vi "writeToXML.vi"(8 "error in (no error)":errorcluster, 10 "Class Label":string, 11 "ADCPointingCorrectionOffsets in":refnum<class "ADCPointingCorrectionOffsets.lvclass">) -> (0 "error out":errorcluster, 2 "XML out":string, 3 "ADCPointingCorrectionOffsets out":refnum<class "ADCPointingCorrectionOffsets.lvclass">)   [LabVIEW 2022 SP3, in "TCSDataDefinitions.lvlib" / "TCSAtmosphericDispersionCommand.lvlib" / "ADCPointingCorrectionOffsets.lvclass"]
uses:
  ADCPointingCorrectionOffsets.lvclass
  <userlib>/Common/UnitsAndXML/FlattenItemWithUnitToXML/FlattenPlaneAngleToXML/PlaneAngleUnit.ctl
  ADCPointingCorrectionOffsets.lvclass/ADCPointingCorrectionOffsets.ctl
  TCSAtmosphericDispersionCommand/TCSAtmosphericDispersionCommand.lvclass
  <userlib>/Common/UnitsAndXML/UnitsAndXML.lvlib
  <userlib>/Common/XML/XMLGenerator/XMLGenerator.lvclass
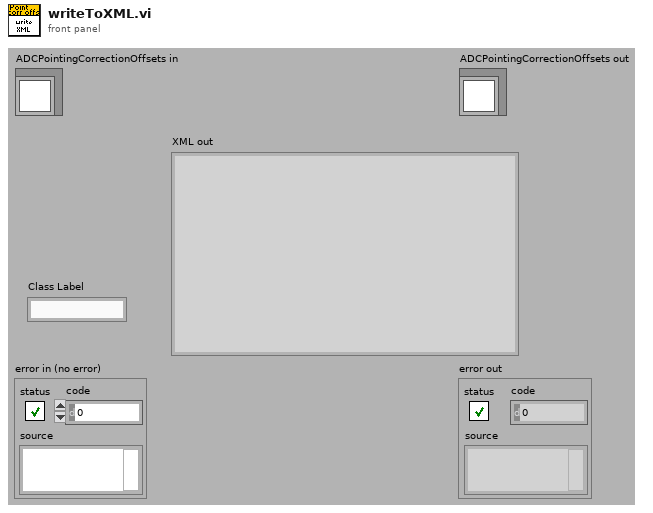
[diagram p1: front panel]
types:
  T1 = typedef "UnitsAndXML.lvlib/PlaneAngleUnit.ctl" = enum16{"rad", "deg", "'", "\""}
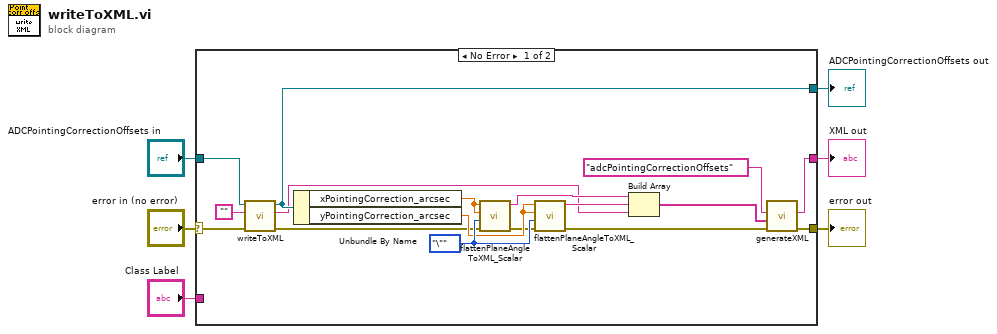
[diagram p0: block diagram]
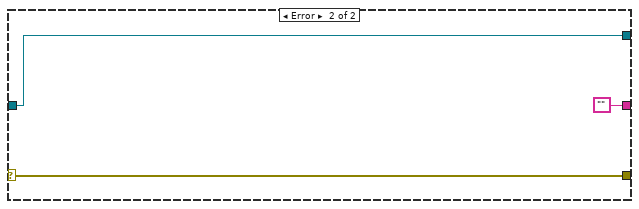
[diagram p2: hidden frame]
diagram:
  n1 = case shown="No Error" "error in (no error)" {
    selector: "error in (no error)" -> [w9 w26]
    tunnel: [w8 w26] -> w5
    tunnel: [w21 w25] -> w3
    tunnel: "ADCPointingCorrectionOffsets in" -> [w23 w25]
    tunnel: [w7 ""] -> w2
    tunnel: "Class Label" -> [_ _]
    frame No Error {
      w19 = PlaneAngleUnit."\"" ("planeAngleUnitInXML")
      n2 = call-parent "writeToXML.vi"("error in (no error)"=w9, "ClassLabel"="", "TCSAtmosphericDispersionCommand in"=w23) -> ("error out"=w17:errorcluster, "XML out"=w13:string, "TCSAtmosphericDispersionCommand out"=w21:refnum<class "ADCPointingCorrectionOffsets.lvclass">)  [unwired: 6 in]
      n3 = Unbundle By Name(w21) -> ("xPointingCorrection_arcsec"=w20:dbl[unit], "yPointingCorrection_arcsec"=w18:dbl[unit])
      n4 = call <userlib>:"flattenPlaneAngleToXML_Scalar.vi"("error in (no error)"=w17, "planeAngleUnitInXML"=w19, "planeAngleAgain"=w20, "planeAngle"=w20) -> ("error out"=w16:errorcluster, "xmlString"=w15:string)  [unwired: 6 in]
      n5 = call <userlib>:"flattenPlaneAngleToXML_Scalar.vi"("error in (no error)"=w16, "planeAngleUnitInXML"=w19, "planeAngleAgain"=w18, "planeAngle"=w18) -> ("error out"=w10:errorcluster, "xmlString"=w14:string)  [unwired: 6 in]
      n6 = Build Array(w15, w14, w13) -> (w12:string[])
      n7 = call <userlib>:"generateXML.vi"("error in"=w10, "childrenXML"=w12, "elementName"="adcPointingCorrectionOffsets" ("Class Label")) -> ("error out"=w8:errorcluster, "XML out"=w7:string)  [unwired: 6 in, 1 out]
    }
    frame Error {
    }
  }
  "error out" <- w5
  "ADCPointingCorrectionOffsets out" <- w3
  "XML out" <- w2
